vi "Special 2 Step 3 (SubVI).vi"(0 "Ldist":dbl, 5 "lbrc":dbl, 7 "aLB":dbl, 9 "aLB1":dbl, 11 "aLB2":dbl) -> (4 "lcx1":dbl, 6 "lcy1":dbl, 8 "rcx1":dbl, 10 "rcy1":dbl, 15 "aLB1+aLB2":dbl)   [LabVIEW 2015]
uses:
  <vilib>/express/express arith-compare/Formula/XNode/ExpressFormulaBlockNode.xnode
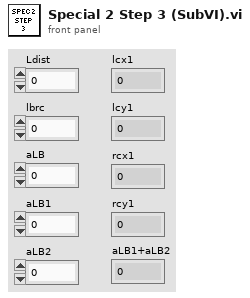
[diagram p1: front panel]
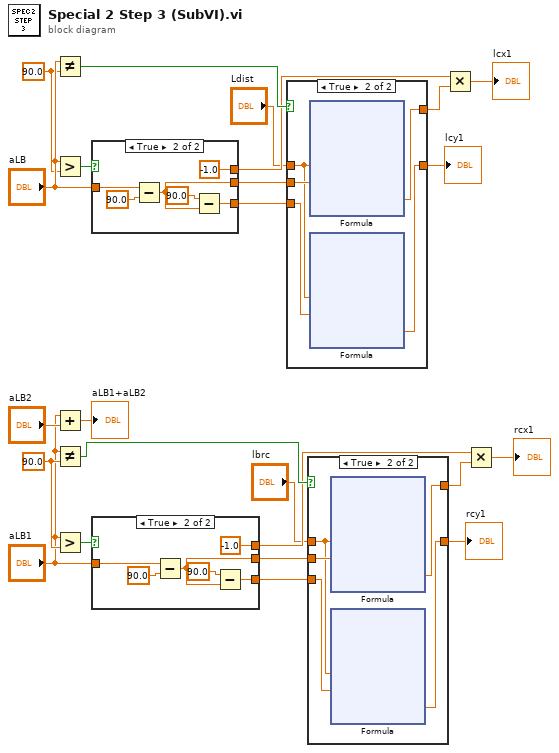
[diagram p0: block diagram]
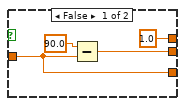
[diagram p2: hidden frame]
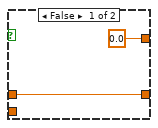
[diagram p3: hidden frame]
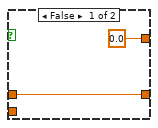
[diagram p4: hidden frame]
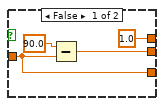
[diagram p5: hidden frame]
diagram:
  w17 = 90.0 ("y")
  w18 = 90.0 ("y")
  n1 = Not Equal?(x="aLB", y=w18) -> (x != y?=w21:bool)
  n2 = Greater?(x="aLB", y=w18) -> (0:w22:bool)
  n3 = Add(x="aLB1", y="aLB2") -> (x+y=→"aLB1+aLB2":dbl)
  n4 = Not Equal?(x="aLB1", y=w17) -> (x != y?=w20:bool)
  n5 = Greater?(x="aLB1", y=w17) -> (0:w8:bool)
  n6 = case shown="True" w22 {
    tunnel: "aLB" -> [w26 w34]
    tunnel: [w27 w31] -> w15
    tunnel: [w26 w30] -> w16
    tunnel: [1.0 -1.0] -> w11
    frame False {
      n7 = Subtract(x=90.0, y=w26) -> (x-y=w27:dbl)
    }
    frame True {
      n8 = Subtract(x=w34, y=90.0) -> (x-y=w31:dbl)
      n9 = Subtract(x=90.0, y=w31) -> (x-y=w30:dbl)
    }
  }
  n10 = case shown="True" w8 {
    tunnel: "aLB1" -> [w36 w44]
    tunnel: [w37 w41] -> w13
    tunnel: [w36 w40] -> w14
    tunnel: [1.0 -1.0] -> w10
    frame False {
      n11 = Subtract(x=90.0, y=w36) -> (x-y=w37:dbl)
    }
    frame True {
      n12 = Subtract(x=w44, y=90.0) -> (x-y=w41:dbl)
      n13 = Subtract(x=90.0, y=w41) -> (x-y=w40:dbl)
    }
  }
  n14 = case shown="True" w21 {
    tunnel: w16 -> [_ w51]
    tunnel: w15 -> [_ w50]
    tunnel: [0.0 ("Result") w49] -> w12
    tunnel: [w46 w48] -> w3
    tunnel: "Ldist" -> [w46 w47]
    frame False {
    }
    frame True {
      n15 = xnode "Formula"("Ldist"=w47, "aRX"=w50) -> ("Result"=w49:dbl)  [unwired: 1 in, 1 out]
      n16 = xnode "Formula"("Ldist"=w47, "aRY"=w51) -> ("Result"=w48:dbl)  [unwired: 1 in, 1 out]
    }
  }
  "lcy1" <- w3
  n17 = case shown="True" w20 {
    tunnel: w14 -> [_ w78]
    tunnel: w13 -> [_ w77]
    tunnel: [0.0 ("Result") w76] -> w9
    tunnel: [w73 w75] -> w5
    tunnel: "lbrc" -> [w73 w74]
    frame False {
    }
    frame True {
      n18 = xnode "Formula"("lbrc"=w74, "aRX"=w77) -> ("Result"=w76:dbl)  [unwired: 1 in, 1 out]
      n19 = xnode "Formula"("lbrc"=w74, "aRY"=w78) -> ("Result"=w75:dbl)  [unwired: 1 in, 1 out]
    }
  }
  "rcy1" <- w5
  n20 = Multiply(x=w11, y=w12) -> (x*y=→"lcx1":dbl)
  n21 = Multiply(x=w10, y=w9) -> (x*y=→"rcx1":dbl)
